vi "Set Enable State on Multiple Controls.vi"(8 "Error In":errorcluster, 10 "Disabled State":T1(ring), 11 "Controls":refnum<vi>[](array[refnum])) -> (0 "Error Out":errorcluster)   [LabVIEW 2014]
doc: "Sets all the controls in the input array to the \"Enable state\" value."
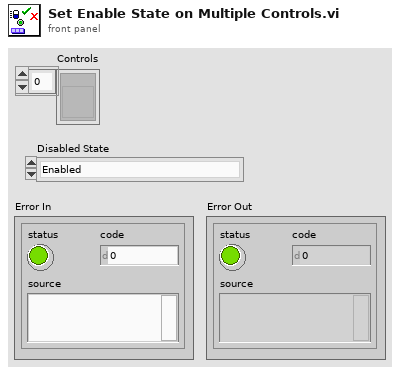
[diagram p1: front panel]
types:
  T1 = enum8{"Enabled", "Disabled", "Disabled and Grayed Out"}
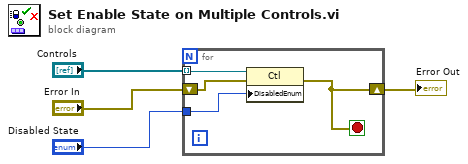
[diagram p0: block diagram]
diagram:
  n1 = for {
    tunnel: "Controls" -> [w8] mode=indexing
    tunnel: "Disabled State" -> [w7]
    shift-right: [w5] -> w3
    shift-left: "Error In" -> [w6]
    stop <- w5 stop-if-true
    n2 = property class="Ctl"(reference=w8, error in=w6, "DisabledEnum"=w7) -> (error out=w5:errorcluster)  [unwired: 1 out]
  }
  "Error Out" <- w3
